vi "serial read v3.vi"() -> ()   [LabVIEW 2023]
uses:
  <vilib>/Instr/_visa.llb/VISA Configure Serial Port (Instr).vi
panel:
  out "VISA resource name out":refnum<visa-resource-name>
  out "return count":u32
  out "concatenated string":string
  in  "Slide 2":dbl(slide) scale=0.0..1000.0
  in  "write buffer":string
  in  "baud rate":u32=9600
  out "read buffer":string
  out "Loop Number":i32
  in  "stop":bool
  in  "COM":refnum<visa-resource-name>
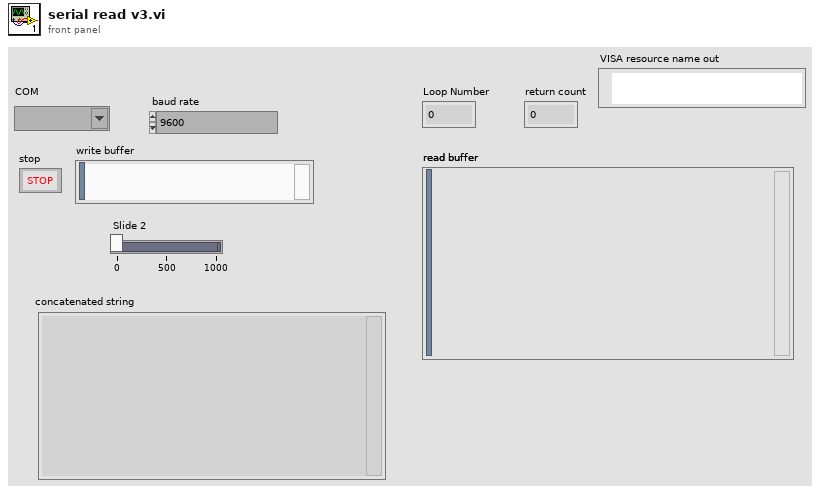
[diagram p1: front panel]
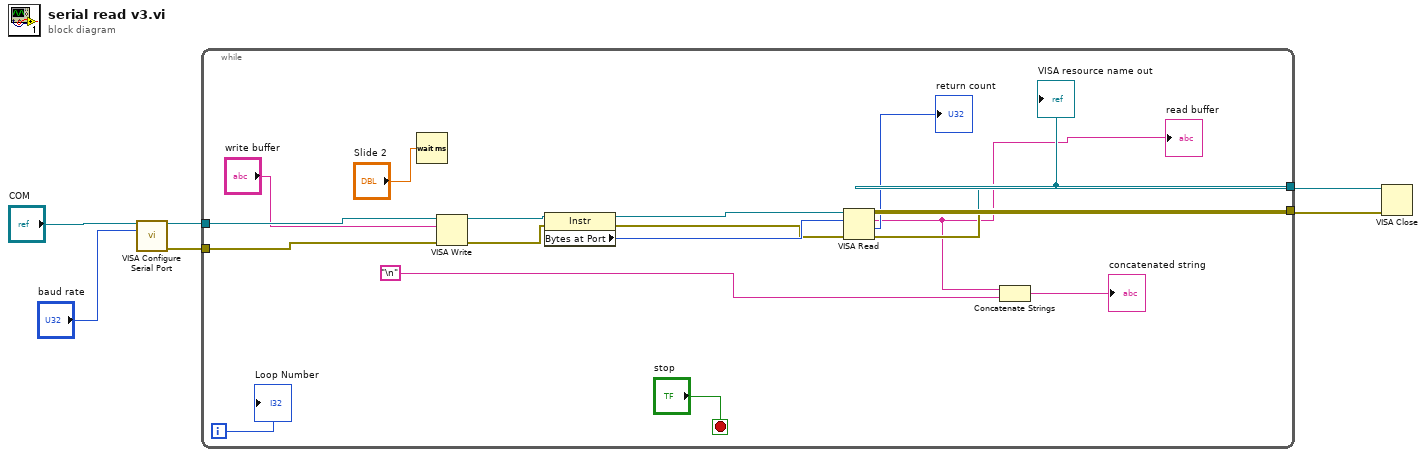
[diagram p0: block diagram]
diagram:
  n1 = call-poly "VISA Configure Serial Port"("VISA resource name"="COM", "baud rate (9600)"="baud rate") -> ("VISA resource name out"=w5:refnum<visa-resource-name>, "error out"=w6:errorcluster)  [unwired: 12 in]
  n2 = while {
    tunnel: w6 -> [w20]
    tunnel: w5 -> [w21]
    tunnel: [w19] -> w2
    tunnel: [w18] -> w1
    i -> [w22]
    stop <- "stop" stop-if-true
    n3 = Wait (ms)(milliseconds to wait="Slide 2") -> ()  [unwired: 1 out]
    n4 = VISA Write(VISA resource name=w21, write buffer="write buffer", error in (no error)=w20) -> (VISA resource name out=w12:refnum<visa-resource-name>, error out=w11:errorcluster)  [unwired: 1 out]
    n5 = property class="Instr"(reference=w12, error in=w11) -> (reference out=w10:refnum<visa-resource-name>, error out=w8:errorcluster, "Bytes at Port"=w9:u32)
    n6 = VISA Read(VISA resource name=w10, byte count=w9, error in (no error)=w8) -> (VISA resource name out=w19:refnum<visa-resource-name>, read buffer=w7:string, return count=→"return count":u32, error out=w18:errorcluster)
    "read buffer" <- w7
    "VISA resource name out" <- w19
    n7 = Concatenate Strings(w7, "\n") -> (→"concatenated string":string)
    "Loop Number" <- w22
  }
  n8 = VISA Close(VISA resource name=w2, error in (no error)=w1) -> ()  [unwired: 1 out]
